vi "PIM Select Instruments to Use.vi"(6 "Driver Ref (null)":T1, 7 "PIM Test Parameters":T2={"Stimulus"={"C1 Pwr dBm"=0.0, "C2 Pwr dBm"=0.0, "Power Units"=enum."dBm", "Meas Type"=enum."Time", "C1 Freq MHz"=0.0, "C2 Freq MHz"=0.0, "Swept Freq Step"=0}, "Measure"={"IM Order"=0, "Direction"=0, "Averaging"=1, "ALC ON?"=TRUE, "Peak Hold?"=TRUE, "Peak last N"=1, "Ref Level dBm"=-100.0, "Ref Units"=enum."dBm", "Num Samples"=1, "Sample units"=enum."Sample(s)", "Update Rate (s)"=0.0, "DUT PORT"=enum."Port 1", "Percent (%)"=100}, "Display"={"Power Scale"={"yRange_min"=0, "yRange_max"=0}, "xRange_span"=5}} {"Stimulus"."Swept Freq Step" items=[".2", ".4", "1.0", "2.0"]; "Measure"."Averaging" items=["None", "Minimum", "Normal", "High", "Maximum"]; "Measure"."Direction" items=["Reverse", "Forward", "Auxiliary"]; "Measure"."IM Order" items=["3rd", "5th", "7th", "9th", "11th", "13th", "15th", "17th", "19th", "21st", "23rd", "25th", "27th", "29th", "31st", "33rd"]}, 9 "error in (no error)":errorcluster, 10 "Available Instruments":T12[](array[typedef])) -> (1 "error out":errorcluster, 2 "Selected Instrument":T12, 4 "Driver Ref out":T1)   [LabVIEW 2011]
uses:
  typedefs/Instrument Record.ctl
  TypeDefs/PIM Test Parameters.ctl
  TypeDefs/PIM Stimulus Parameters.ctl
  BPIMCore/HW IO/PIM Sweep Step Size.ctl
  TypeDefs/PIM Measurement Parameters.ctl
  BPIMCore/HW IO/IMOrder.ctl
  BPIMCore/HW IO/MeasMode.ctl
  BPIMCore/HW IO/HW Averaging.ctl
  TypeDefs/PIM Meas Units.ctl
  BPIMCore/HW IO/DUTport.ctl
  TypeDefs/PIM Display Parameters.ctl
  drivers/PIM/PIM Driver Ref.ctl
  drivers/PIM/PIM Command.ctl
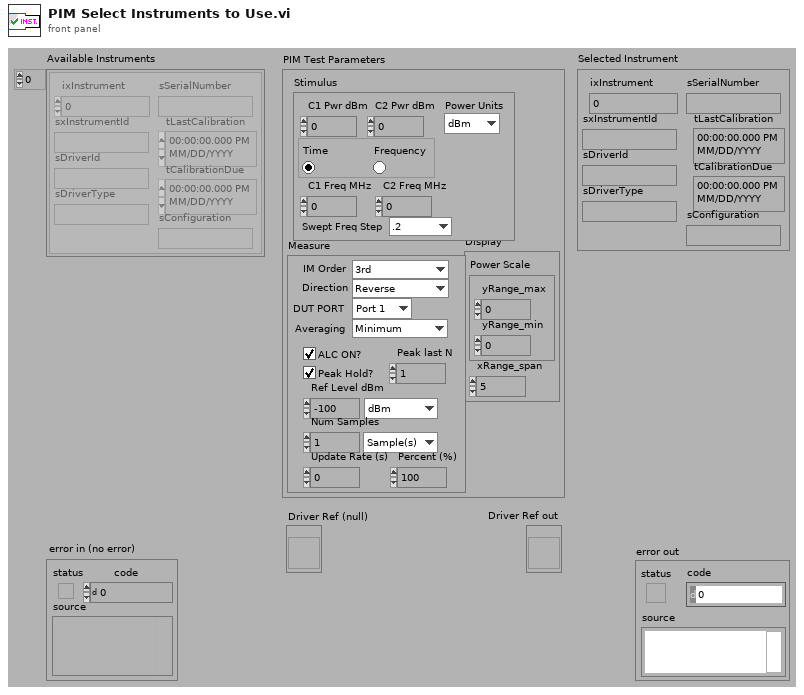
[diagram p1: front panel]
types:
  T1 = typedef "PIM Driver Ref.ctl" = refnum<vi>
  T2 = typedef "PIM Test Parameters.ctl" = cluster{"Stimulus":T3, "Measure":T5, "Display":T11}
  T3 = typedef "PIM Stimulus Parameters.ctl" = cluster{"C1 Pwr dBm":dbl, "C2 Pwr dBm":dbl, "Power Units":enum16{"dBm", "Watts"}, "Meas Type":enum32{"Time", "Frequency"}, "C1 Freq MHz":dbl, "C2 Freq MHz":dbl, "Swept Freq Step":T4}
  T4 = typedef "PIM Sweep Step Size.ctl" = u16
  T5 = typedef "PIM Measurement Parameters.ctl" = cluster{"IM Order":T6, "Direction":T7, "Averaging":T8, "ALC ON?":bool, "Peak Hold?":bool, "Peak last N":u32, "Ref Level dBm":dbl, "Ref Units":enum16{"dBm", "dBc"}, "Num Samples":u32, "Sample units":T9, "Update Rate (s)":dbl, "DUT PORT":T10, "Percent (%)":u8}
  T6 = typedef "IMOrder.ctl" = u8
  T7 = typedef "MeasMode.ctl" = u16
  T8 = typedef "HW Averaging.ctl" = u16
  T9 = typedef "PIM Meas Units.ctl" = enum16{"Sample(s)", "Second(s)", "Sweep(s)"}
  T10 = typedef "DUTport.ctl" = enum16{"Port 1", "Port 2"}
  T11 = typedef "PIM Display Parameters.ctl" = cluster{"Power Scale":cluster{"yRange_min":i32, "yRange_max":i32}, "xRange_span":u32}
  T12 = typedef "Instrument Record.ctl" = cluster{"ixInstrument":i32, "sxInstrumentId":string, "sDriverId":string, "sDriverType":string, "sSerialNumber":string, "tLastCalibration":timestamp, "tCalibrationDue":timestamp, "sConfiguration":string}
  T13 = typedef "PIM Command.ctl" = enum16{"LOAD", "KEEP ALIVE", "VALIDATE", "INITIALIZE", "PRESET", "GET CALIBRATION", "SET STIMULUS", "TOGGLE TX POWER", "SET TX ON", "SET TX OFF", "MEASURE", "UNLOAD"}
  T14 = typedef "PIM Stimulus.ctl" = cluster{"Carrier Frequencies":cluster{"C1 Freq, MHz":dbl, "C2 Freq, MHz":dbl}, "Carrier Powers":cluster{"C1 Power,dBm":dbl, "C2 Power, dBm":dbl}, "Measurement Parameters":T15, "Measurement Setup":cluster{"Meas Type":enum32{"Time", "Frequency"}, "TXStep":T4}}
  T15 = typedef "PIM Cmd Params.ctl" = cluster{"IM Order":T6, "Averaging":T8, "Direction":T7, "Enable ALC?":bool, "Enable SingleIM?":bool, "Display Units":T16, "VA Hold?":bool, "DUT PORT":T10}
  T16 = typedef "display_unit_format.ctl" = enum16{"dBm", "dBc"}
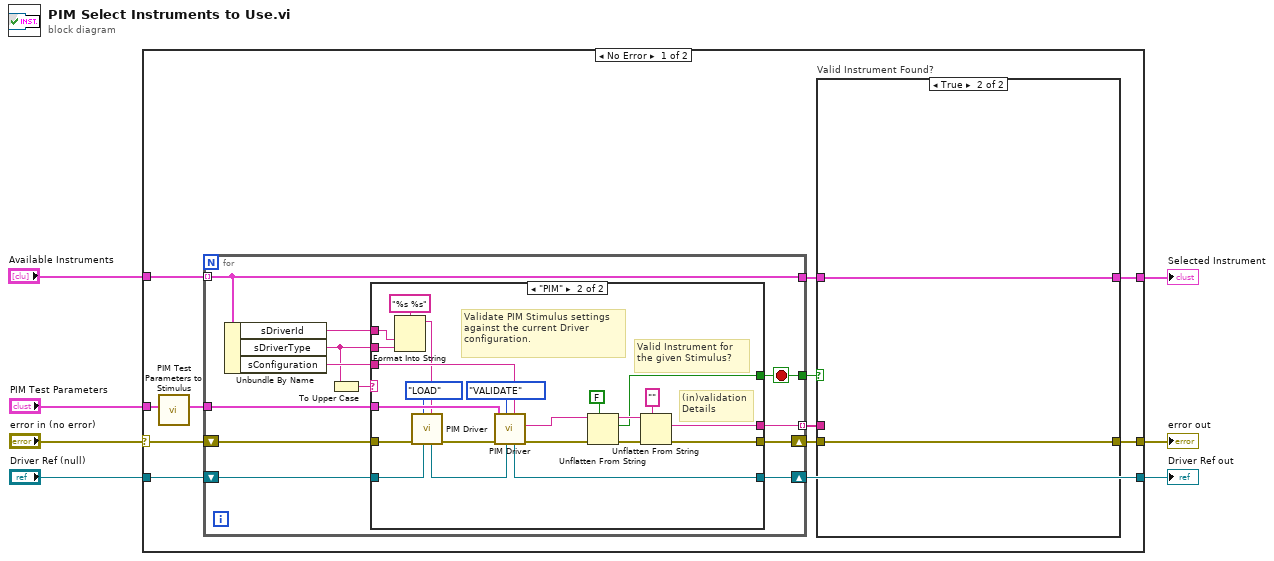
[diagram p0: block diagram]
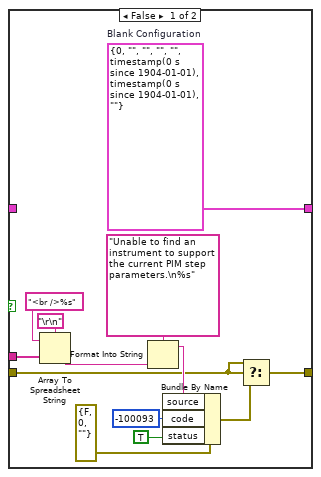
[diagram p2: hidden frame]
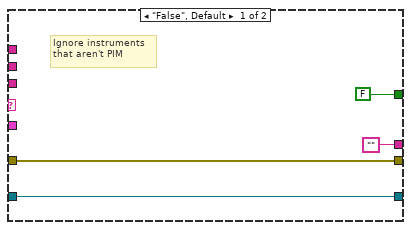
[diagram p3: hidden frame]
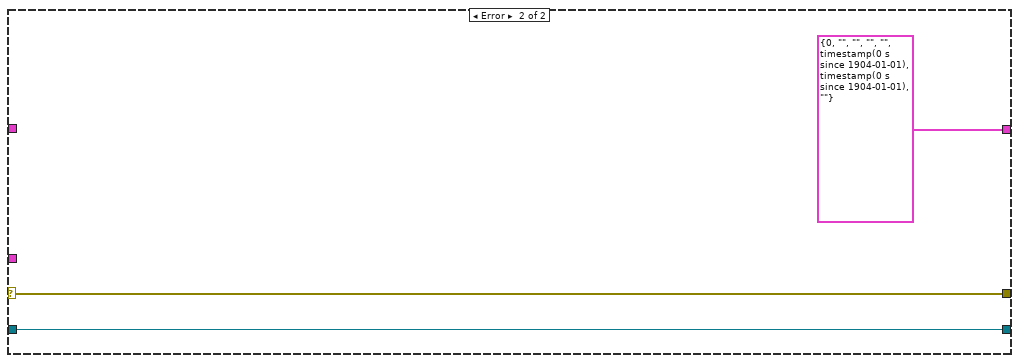
[diagram p4: hidden frame]
diagram:
  n1 = case shown="No Error" "error in (no error)" {
    selector: "error in (no error)" -> [w8 w75]
    tunnel: "PIM Test Parameters" -> [w19 _]
    tunnel: "Driver Ref (null)" -> [w17 w74]
    tunnel: "Available Instruments" -> [w16 _]
    tunnel: [w13 T12 {"ixInstrument"=0, "sxInstrumentId"="", "sDriverId"="", "sDriverType"="", "sSerialNumber"="", "tLastCalibration"=timestamp(0 s since 1904-01-01), "tCalibrationDue"=timestamp(0 s since 1904-01-01), "sConfiguration"=""} ("Instrument Information (Cluster)")] -> w4
    tunnel: [w10 w75] -> w3
    tunnel: [w9 w74] -> w2
    frame No Error {
      n2 = call "PIM Test Parameters to Stimulus.vi"("PIM Test Parameters"=w19) -> ("PIM Measurement Stimulus"=w18:T14)  [unwired: 10 out]
      n3 = for {
        tunnel: w18 -> [w46]
        shift-right: [w40] -> w9
        shift-left: w17 -> [w45]
        shift-right: [w43] -> w12
        shift-left: w8 -> [w44]
        tunnel: w16 -> [w37] mode=indexing
        tunnel: [w39] -> w11 mode=indexing
        tunnel: [w38] -> w15
        tunnel: [w37] -> w14
        stop <- w38 stop-if-true
        n4 = Unbundle By Name(w37) -> ("sDriverId"=w36:string, "sDriverType"=w35:string, "sConfiguration"=w42:string)
        n5 = To Upper Case(1:w35) -> (0:w41:string)
        n6 = case shown="\"PIM\"" w41 {
          tunnel: w46 -> [_ w72]
          tunnel: w45 -> [w50 w59]
          tunnel: w44 -> [w49 w61]
          tunnel: [w49 w63] -> w43
          tunnel: w42 -> [_ w70]
          tunnel: [w50 w69] -> w40
          tunnel: [FALSE ("Boolean") w64] -> w38
          tunnel: ["" w62] -> w39
          tunnel: w36 -> [_ w55]
          tunnel: w35 -> [_ w54]
          frame "False", Default {
            # "Ignore instruments that aren't PIM"
          }
          frame "PIM" {
            # "(in)validation\nDetails"
            # "Valid Instrument for the given Stimulus?"
            # "Validate PIM Stimulus settings against the current Driver configuration."
            n7 = Format Into String(format string="%s %s", w55, w54) -> (resulting string=w53:string)  [unwired: 2 in, 1 out]
            n8 = call "PIM Driver.vi"("PIM Driver Name/Configuration"=w53, "Driver Ref (null)"=w59, "PIM Command"=PIM_Command."LOAD", "error in (no error)"=w61) -> ("error out"=w60:errorcluster, "duplicate driver ref"=w58:T1)  [unwired: 1 in, 5 out]
            n9 = call "PIM Driver.vi"("PIM Driver Name/Configuration"=w70, "Driver Ref (null)"=w58, "PIM Command"=PIM_Command."VALIDATE", "error in (no error)"=w60, "Stimulus"=w72) -> ("error out"=w51:errorcluster, "Variant Output"=w52:string, "duplicate driver ref"=w69:T1)  [unwired: 4 out]
            n10 = Unflatten From String(type=FALSE ("Boolean"), binary string=w52, error in (no error)=w51) -> (rest of the binary string=w65:string, value=w64:bool, error out=w66:errorcluster)  [unwired: 2 out]
            n11 = Unflatten From String(type="" ("data string"), binary string=w65, error in (no error)=w66) -> (value=w62:string, error out=w63:errorcluster)  [unwired: 3 out]
          }
        }
      }
      n12 = case "Valid Instrument Found?" shown="True" w15 {
        tunnel: w14 -> [_ w34]
        tunnel: [w32 w34] -> w13
        tunnel: w12 -> [w22 w33]
        tunnel: w11 -> [w28 _]
        tunnel: [w20 w33] -> w10
        frame False {
          w32 = T12 {"ixInstrument"=0, "sxInstrumentId"="", "sDriverId"="", "sDriverType"="", "sSerialNumber"="", "tLastCalibration"=timestamp(0 s since 1904-01-01), "tCalibrationDue"=timestamp(0 s since 1904-01-01), "sConfiguration"=""}  # Blank Configuration
          n13 = Array To Spreadsheet String(delimiter (Tab)="\r\n", array=w28, 3:"<br />%s" ("format string")) -> (spreadsheet string=w25:string)
          n14 = Format Into String(format string="Unable to find an instrument to support the current PIM step parameters.\n%s" ("source"), w25) -> (resulting string=w29:string)  [unwired: 2 in, 1 out]
          n15 = Bundle By Name(cluster=errorcluster {"status"=FALSE, "code"=0, "source"=""} ("error IO"), "source"=w29, "code"=-100093, "status"=TRUE) -> (w21:errorcluster)
          n16 = Select(t=w22, s=w22, f=w21) -> (s? t:f=w20:errorcluster)
        }
        frame True {
        }
      }
    }
    frame Error {
    }
  }
  "Selected Instrument" <- w4
  "error out" <- w3
  "Driver Ref out" <- w2
